vi "Pump Relay Test.vi"(8 "error in (no error)":errorcluster, 10 "Message IN":string) -> (0 "error out":errorcluster, 1 "Result (bool)":bool, 2 "Message OUT":string, 3 "VISA resource name 2":refnum<visa-resource-name>)   [LabVIEW 2022 SP3]
panel:
  in  "FAIL":bool
  in  "PASS":bool
  in  "Pump Contactor":bool
  out "Result (color)":u32(colorbox)
  # "Toggle the pump contactor. Does it open and close as expected?"
  # "Off = Open\nOn = Closed"
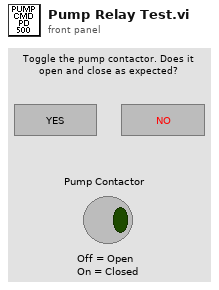
[diagram p1: front panel]
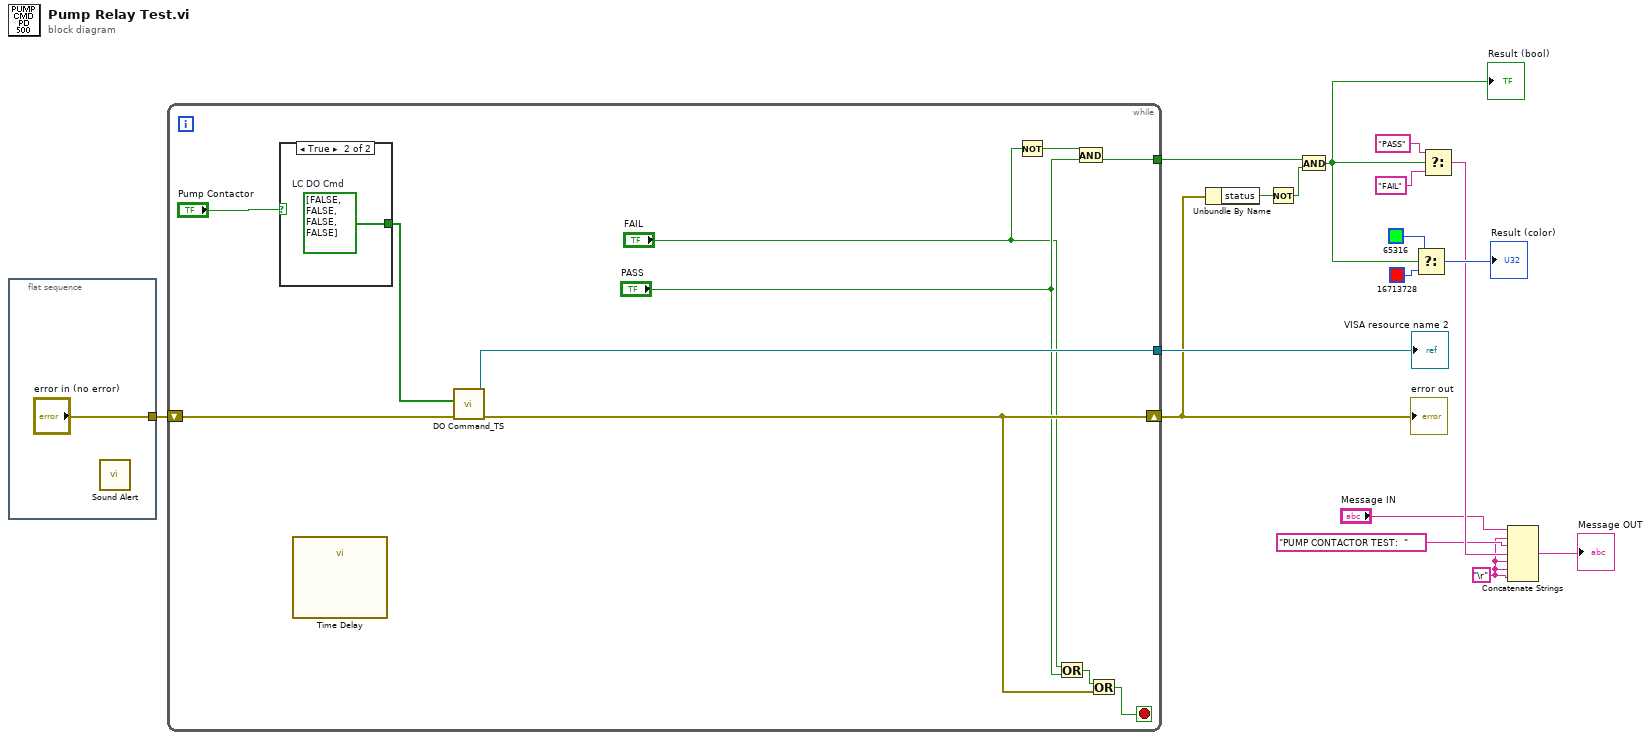
[diagram p0: block diagram]
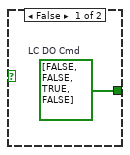
[diagram p2: hidden frame]
diagram:
  w3 = "\r"
  n1 = flat-sequence {
    tunnel: ["error in (no error)"] -> w14
    frame #0 {
      n2 = call "Sound Alert.vi"() -> ()  [unwired: 12 in]
    }
  }
  n3 = while {
    shift-right: [w26] -> w1
    shift-left: w14 -> [w29]
    tunnel: [w28] -> w17
    tunnel: [w22] -> w2
    stop <- w24 stop-if-true
    n4 = case shown="True" "Pump Contactor" {
      tunnel: [w30 w31] -> w19
      frame False {
        w30 = bool[] [FALSE, FALSE, TRUE, FALSE]  # LC DO Cmd
      }
      frame True {
        w31 = bool[] [FALSE, FALSE, FALSE, FALSE]  # LC DO Cmd
      }
    }
    n5 = call "Time Delay"() -> ()  [unwired: 11 in, 1 out]
    n6 = call "DO Command_TS.vi"("error in (no error)"=w29, "DO Command"=w19) -> ("error out"=w26:errorcluster, "VISA Refnum out"=w28:refnum<visa-resource-name>)  [unwired: 8 in]
    n7 = Not(x="FAIL") -> (.not. x?=w21:bool)
    n8 = Or(x="FAIL", y="PASS") -> (x .or. y?=w25:bool)
    n9 = And(x=w21, y="PASS") -> (x .and. y?=w22:bool)
    n10 = Or(x=w25, y=w26) -> (x .or. y?=w24:bool)
  }
  "error out" <- w1
  "VISA resource name 2" <- w17
  n11 = Unbundle By Name(w1) -> ("status"=w10:bool)
  n12 = Not(x=w10) -> (.not. x?=w9:bool)
  n13 = And(x=w2, y=w9) -> (x .and. y?=w8:bool)
  "Result (bool)" <- w8
  n14 = Select(t=u32 65316 ("Result (color)"), s=w8, f=u32 16713728 ("Result (color)")) -> (s? t:f=→"Result (color)":u32)
  n15 = Select(t="PASS", s=w8, f="FAIL") -> (s? t:f=w6:string)
  n16 = Concatenate Strings("Message IN", w3, "PUMP CONTACTOR TEST:  ", w6, w3, w3, w3) -> (→"Message OUT":string)
